vi "Temp - Change Font.vi"(8 "error in (no error)":errorcluster, 9 "message font.Text.Justification":enum16{"Left", "Center", "Right"}(ring), 10 "message font.Text.Font Size":u32=30) -> (0 "error out":errorcluster, 3 "Theme out":refnum<class "Theme.lvclass">)   [LabVIEW 2021, in "Theme.lvclass"]
doc: "Change the font of the pop-ups \n\n<b>Code Developed By:</b> +\nDaniel Coons +\nhttps://github.com/danielcoons/tsc-pop-up"
uses:
  Theme.lvclass
  Theme.lvclass/Theme.ctl
  Popup/PopUp Theme Global.vi
  Popup/Popup.lvclass
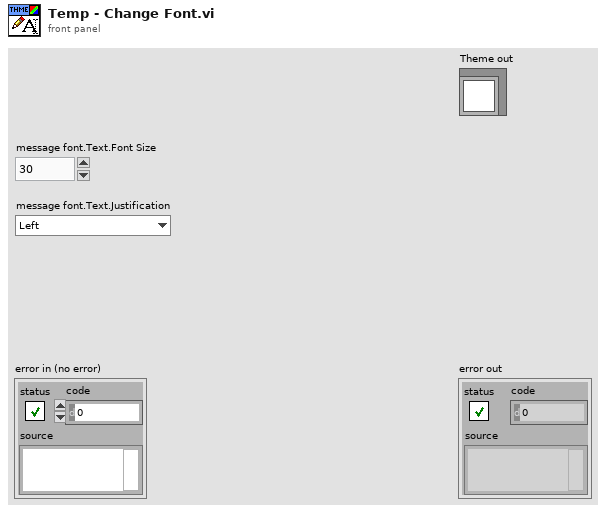
[diagram p1: front panel]
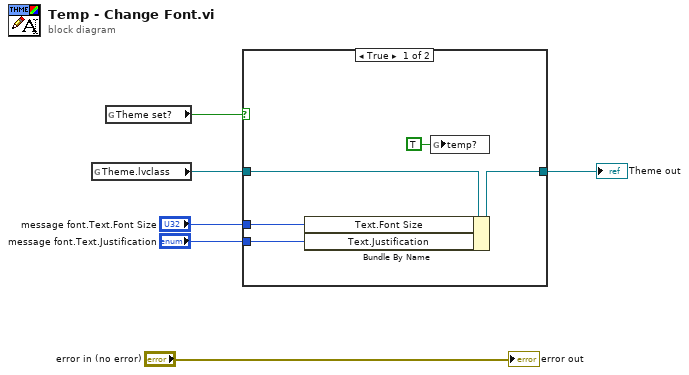
[diagram p0: block diagram]
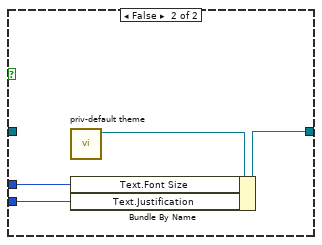
[diagram p2: hidden frame]
diagram:
  n1 = global read "PopUp Theme Global.vi" "Theme.lvclass"() -> (w4:refnum<class "Theme.lvclass">)
  n2 = global read "PopUp Theme Global.vi" "Theme set?"() -> (w5:bool)
  n3 = case shown="True" w5 {
    tunnel: w4 -> [w11 _]
    tunnel: "message font.Text.Font Size" -> [w10 w15]
    tunnel: "message font.Text.Justification" -> [w9 w14]
    tunnel: [w8 w13] -> w1
    frame True {
      n4 = Bundle By Name(cluster=w11, "Text.Font Size"=w10, "Text.Justification"=w9) -> (w8:refnum<class "Theme.lvclass">)
      n5 = global write "PopUp Theme Global.vi" "temp?"(TRUE ("temp?")) -> ()
    }
    frame False {
      n6 = call "priv-default theme.vi"() -> ("Theme out"=w12:refnum<class "Theme.lvclass">)  [unwired: 11 in]
      n7 = Bundle By Name(cluster=w12, "Text.Font Size"=w15, "Text.Justification"=w14) -> (w13:refnum<class "Theme.lvclass">)
    }
  }
  "Theme out" <- w1
  "error out" <- "error in (no error)"
